vi "PoseAndTargeting.vi"() -> ()   [LabVIEW 2023]
doc: "Manages the robot's pose (position, heading, and velocity) and targeting information. Data from the IMU, swerve drive encoders, swerve azimuth encoders, turret enoder, and LimeLight are fused together to estimate these values. Supports pose resets on boot, from the Autonomous Sequencer, and on command from the FRC 4265 Dashboard."
uses:
  GlobalDrivebase.vi
panel:
  in  "Using 3D Targeting":bool=TRUE
  in  "Max Vision X (in)":dbl=200.0
  in  "Min Timed Aligned (ms)":u32=200
  in  "Acceptable Heading Error (deg)":dbl=5.0
  in  "Vision Trust Threshold (in)":dbl=10.0
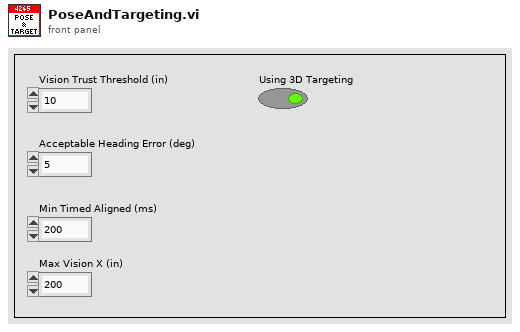
[diagram p1: front panel]
types:
  T1 = cluster{"Transitioning":bool, "Position (in)":dbl, "Velocity (ft/s)":dbl, "Azimuth Position (deg) [-180,+180]":dbl}
  T2 = enum16{"Normal", "Auto Set", "Reset IMU", "Manual Push", "Init"}
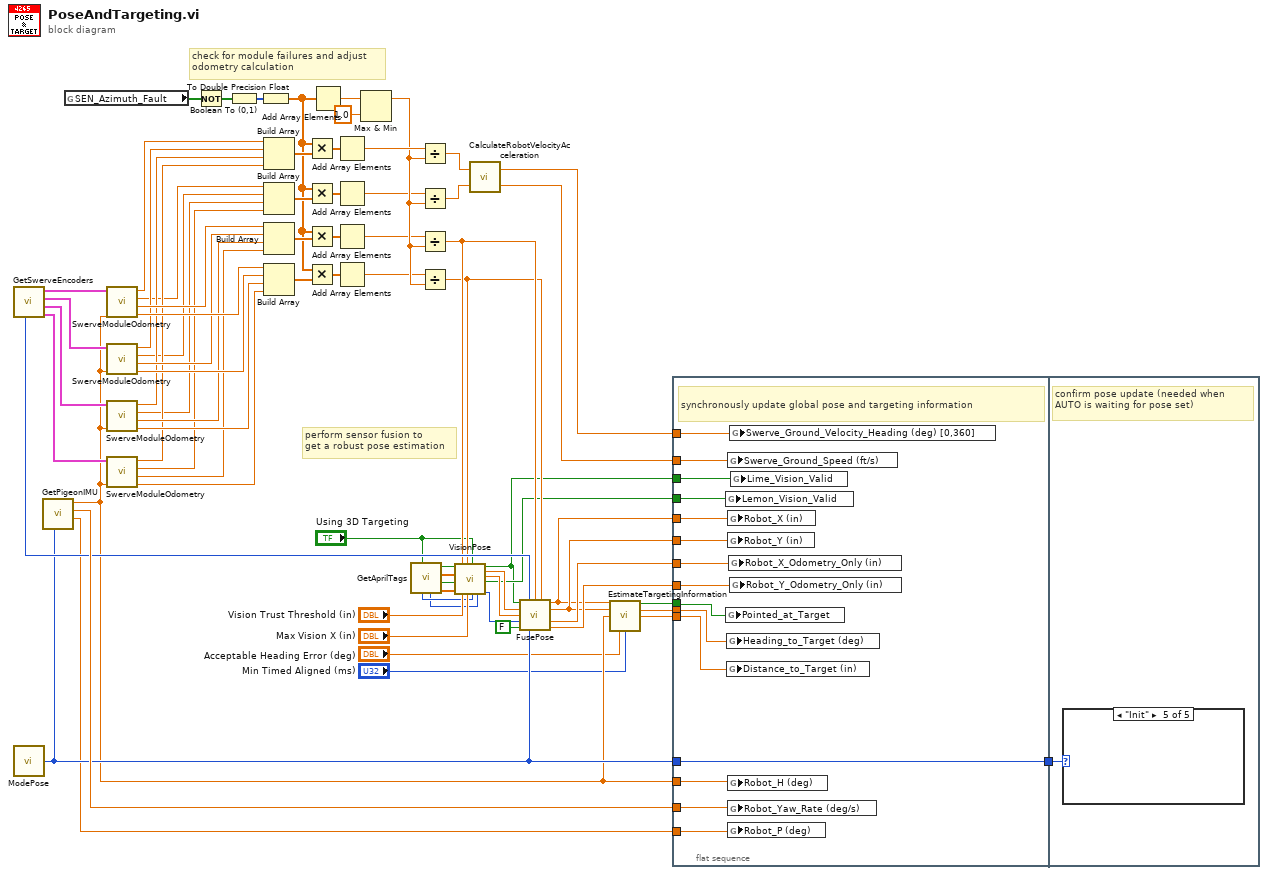
[diagram p0: block diagram]
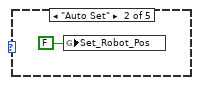
[diagram p3: hidden frame]
diagram:
  # "perform sensor fusion to\nget a robust pose estimation"
  # "check for module failures and adjust\nodometry calculation"
  n1 = call "GetSwerveEncoders.vi"() -> ("Swerve 3 Encoder Data"=w32:T1, "Swerve 2 Encoder Data"=w33:T1, "Swerve 1 Encoder Data"=w34:T1, "Swerve 0 Encoder Data"=w35:T1, "Odometry Timestamp (ms)"=w31:u32)  [unwired: 5 in]
  n2 = call "ModePose.vi"() -> ("Pose Mode"=w27:T2)  [unwired: 1 in]
  n3 = call "GetPigeonIMU.vi"("Pose Mode"=w27) -> ("Yaw (deg)"=w26:dbl, "Yaw Rate (deg/s)"=w56:dbl, "Pitch (deg)"=w22:dbl)  [unwired: 5 in]
  n4 = global read "GlobalDrivebase.vi" "SEN_Azimuth_Fault"() -> (w46:bool[])
  n5 = call "SwerveModuleOdometry.vi"("Robot Heading(deg)"=w26, "Swerve Encoder Data"=w35) -> ("Delta Y (in)"=w72:dbl, "Delta X (in)"=w71:dbl, "Velocity Y (ft/s)"=w64:dbl, "Velocity X (ft/s)"=w53:dbl)  [unwired: 4 in]
  n6 = call "SwerveModuleOdometry.vi"("Robot Heading(deg)"=w26, "Swerve Encoder Data"=w34) -> ("Delta Y (in)"=w73:dbl, "Delta X (in)"=w70:dbl, "Velocity Y (ft/s)"=w63:dbl, "Velocity X (ft/s)"=w67:dbl)  [unwired: 4 in]
  n7 = call "SwerveModuleOdometry.vi"("Robot Heading(deg)"=w26, "Swerve Encoder Data"=w33) -> ("Delta Y (in)"=w74:dbl, "Delta X (in)"=w69:dbl, "Velocity Y (ft/s)"=w62:dbl, "Velocity X (ft/s)"=w66:dbl)  [unwired: 4 in]
  n8 = call "SwerveModuleOdometry.vi"("Robot Heading(deg)"=w26, "Swerve Encoder Data"=w32) -> ("Delta Y (in)"=w75:dbl, "Delta X (in)"=w68:dbl, "Velocity Y (ft/s)"=w61:dbl, "Velocity X (ft/s)"=w65:dbl)  [unwired: 4 in]
  n9 = Not(x=w46) -> (.not. x?=w55:bool[])
  n10 = Boolean To (0,1)(Boolean=w55) -> (0, 1=w54:i16[])
  n11 = To Double Precision Float(number=w54) -> (double precision float=w37:dbl[])
  n12 = Build Array(w53, w67, w66, w65) -> (w47:dbl[])
  n13 = Build Array(w64, w63, w62, w61) -> (w44:dbl[])
  n14 = Build Array(w71, w70, w69, w68) -> (w41:dbl[])
  n15 = Build Array(w72, w73, w74, w75) -> (w38:dbl[])
  n16 = Multiply(x=w37, y=w47) -> (x*y=w52:dbl[])
  n17 = Multiply(x=w37, y=w44) -> (x*y=w45:dbl[])
  n18 = Multiply(x=w37, y=w41) -> (x*y=w42:dbl[])
  n19 = Multiply(x=w37, y=w38) -> (x*y=w39:dbl[])
  n20 = Add Array Elements(numeric array=w37) -> (sum=w50:dbl)
  n21 = Add Array Elements(numeric array=w52) -> (sum=w51:dbl)
  n22 = Add Array Elements(numeric array=w45) -> (sum=w43:dbl)
  n23 = Add Array Elements(numeric array=w42) -> (sum=w40:dbl)
  n24 = Add Array Elements(numeric array=w39) -> (sum=w36:dbl)
  n25 = Max & Min(x=w50, y=1.0) -> (max(x,y)=w48:dbl)  [unwired: 1 out]
  n26 = call "GetAprilTags.vi"("Using 3D Targeting"="Using 3D Targeting") -> ("Lemon AprilTag Data [t-?]"=w4:dbl[], "Lemon Vision Target Valid [t-?]"=w7:bool, "Lime AprilTag Data [t-?]"=w8:dbl[], "Lime Vision Target Valid [t-?]"=w9:bool, "Lemon Vision Timestamp (ms)"=w5:u32, "Lime Vision Timestamp (ms)"=w6:u32)  [unwired: 5 in]
  n27 = Divide(x=w51, y=w48) -> (x/y=w59:dbl)
  n28 = Divide(x=w43, y=w48) -> (x/y=w60:dbl)
  n29 = Divide(x=w40, y=w48) -> (x/y=w15:dbl)
  n30 = Divide(x=w36, y=w48) -> (x/y=w14:dbl)
  n31 = call "VisionPose.vi"("Lime Vision Target Valid [t-?]"=w9, "Lime AprilTag Data [t-?]"=w8, "Lemon Vision Target Valid [t-?]"=w7, "Lemon AprilTag Data [t-?]"=w4, "Odometry Delta X (in) [t0]"=w15, "Vision Trust Threshold (in)"="Vision Trust Threshold (in)", "Odometry Delta Y (in) [t0]"=w14, "Max Vision X (in)"="Max Vision X (in)", "Using 3D Targeting"="Using 3D Targeting", "Lime Vision Timestamp (ms)"=w6, "Lemon Vision Timestamp (ms)"=w5) -> ("Lime Vision Valid [t-?]"=w3:bool, "Combined Vision X (in) [t-?]"=w17:dbl, "Combined Vision Y (in) [t-?]"=w16:dbl, "Lemon Vision Valid [t-?]"=w11:bool, "Lowest Vision Timestamp (ms) [t-?]"=w10:u32)  [unwired: 4 in]
  n32 = call "CalculateRobotVelocityAcceleration.vi"("Velocity Y (ft/s)"=w60, "Velocity X (ft/s)"=w59) -> ("Velocity Magnitude (ft/s)"=w58:dbl, "Velocity Heading (deg)"=w57:dbl)
  n33 = call "FusePose.vi"("Lime Vision Valid [t-?]"=w3, "Odometry Timestamp (ms)"=w31, "Odometry Delta X (in) [t0]"=w15, "Odometry Delta Y (in) [t0]"=w14, "Vision X (in) [t-?]"=w17, "Vision Y (in) [t-?]"=w16, "Vision Timestamp (ms)"=w10, "Lemon Vision Valid [t-?]"=FALSE, "Pose Mode"=w27) -> ("X (in) [t0]"=w18:dbl, "Y (in) [t0]"=w19:dbl, "X Odometry Only (in) [t0]"=w30:dbl, "Y Odometry Only (in) [t0]"=w29:dbl)  [unwired: 3 in]
  n34 = call "EstimateTargetingInformation.vi"("X (in) [t0]"=w18, "Y (in) [t0]"=w19, "Robot Heading (deg)"=w26, "Acceptable Heading Error (deg)"="Acceptable Heading Error (deg)", "Min Timed Aligned (ms)"="Min Timed Aligned (ms)") -> ("Pointed At Target"=w25:bool, "Heading to Target (deg)"=w24:dbl, "Distance to Target (in)"=w23:dbl)  [unwired: 8 in]
  n35 = flat-sequence {
    tunnel: w26 -> [w90]
    tunnel: w11 -> [w89]
    tunnel: w58 -> [w88]
    tunnel: w57 -> [w87]
    tunnel: w56 -> [w86]
    tunnel: w18 -> [w85]
    tunnel: w19 -> [w84]
    tunnel: w30 -> [w83]
    tunnel: w29 -> [w82]
    tunnel: w27 -> [w81]
    tunnel: [w81] -> w28
    tunnel: w25 -> [w79]
    tunnel: w24 -> [w78]
    tunnel: w23 -> [w77]
    tunnel: w22 -> [w80]
    tunnel: w3 -> [w76]
    tunnel: w28 -> [w91]
    frame #0 {
      # "synchronously update global pose and targeting information"
      n36 = global write "GlobalPoseAndTargeting.vi" "Lemon_Vision_Valid"(w89) -> ()
      n37 = global write "GlobalPoseAndTargeting.vi" "Pointed_at_Target"(w79) -> ()
      n38 = global write "GlobalPoseAndTargeting.vi" "Heading_to_Target (deg)"(w78) -> ()
      n39 = global write "GlobalPoseAndTargeting.vi" "Distance_to_Target (in)"(w77) -> ()
      n40 = global write "GlobalPoseAndTargeting.vi" "Swerve_Ground_Speed (ft/s)"(w88) -> ()
      n41 = global write "GlobalPoseAndTargeting.vi" "Robot_X (in)"(w85) -> ()
      n42 = global write "GlobalPoseAndTargeting.vi" "Robot_Y (in)"(w84) -> ()
      n43 = global write "GlobalPoseAndTargeting.vi" "Robot_H (deg)"(w90) -> ()
      n44 = global write "GlobalPoseAndTargeting.vi" "Robot_Yaw_Rate (deg/s)"(w86) -> ()
      n45 = global write "GlobalPoseAndTargeting.vi" "Robot_P (deg)"(w80) -> ()
      n46 = global write "GlobalPoseAndTargeting.vi" "Robot_X_Odometry_Only (in)"(w83) -> ()
      n47 = global write "GlobalPoseAndTargeting.vi" "Swerve_Ground_Velocity_Heading (deg) [0,360]"(w87) -> ()
      n48 = global write "GlobalPoseAndTargeting.vi" "Robot_Y_Odometry_Only (in)"(w82) -> ()
      n49 = global write "GlobalPoseAndTargeting.vi" "Lime_Vision_Valid"(w76) -> ()
    }
    frame #1 {
      # "confirm pose update (needed when AUTO is waiting for pose set)"
      n50 = case shown="\"Init\"" w91 {
        frame "Normal", Default {
        }
        frame "Auto Set" {
          n51 = global write "GlobalPoseAndTargeting.vi" "Set_Robot_Pos"(FALSE ("Set_Robot_Pos")) -> ()
        }
        frame "Reset IMU" {
        }
        frame "Manual Push" {
        }
        frame "Init" {
        }
      }
    }
  }
